vi "temperatura.vi"(9 "error in (no error)":errorcluster, 10 "COM Bluegiga in":refnum<visa-resource-name>) -> (0 "error out":errorcluster, 1 "Numeric":dbl, 2 "Text":string caption="Result", 3 "COM Bluegiga out":refnum<visa-resource-name>)   [LabVIEW 2020]
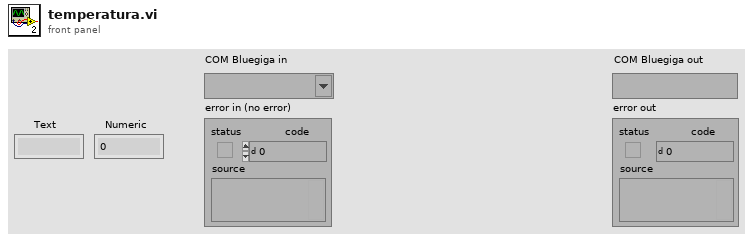
[diagram p1: front panel]
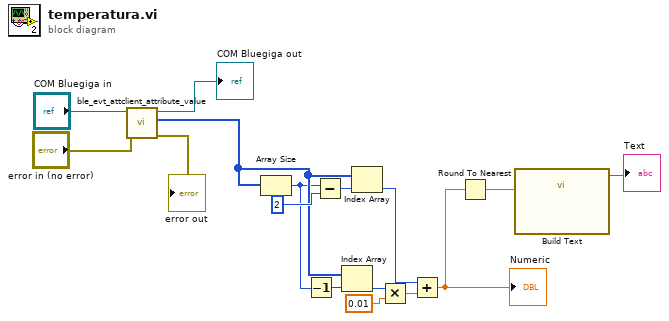
[diagram p0: block diagram]
diagram:
  n1 = call <vilib>:"ble_evt_attclient_attribute_value.vi"("error in (no error)"="error in (no error)", "COM Bluegiga in"="COM Bluegiga in") -> ("error out"=→"error out":errorcluster, "characteristic value"=w13:u8[], "COM Bluegiga out"=→"COM Bluegiga out":refnum<visa-resource-name>)  [unwired: 6 in, 1 out]
  n2 = Array Size(array=w13) -> (size(s)=w11:i32)
  n3 = Decrement(x=w11) -> (x-1=w12:i32)
  n4 = Subtract(x=w11, y=2) -> (x-y=w15:i32)
  n5 = Index Array(array=w13, index=w12) -> (element=w10:u8)
  n6 = Index Array(array=w13, index=w15) -> (element=w7:u8)
  n7 = Multiply(x=w10, y=0.01) -> (x*y=w8:dbl)
  n8 = Add(x=w7, y=w8) -> (x+y=w5:dbl)
  "Numeric" <- w5
  n9 = Round To Nearest(number=w5) -> (nearest integer value=w6:dbl)
  n10 = call "Build Text"("T"=w6) -> ("Result"=→"Text":string)  [unwired: 13 in, 1 out]
